vi "StartRotation.vi"(0 "Graphics Refnum in":refnum<k24>, 1 "X-In":sgl, 2 "Y-In":sgl, 3 "Width-In":sgl, 4 "Height-In":sgl, 5 "error in (no error)":errorcluster, 9 "Rotation(Deg)":sgl) -> (11 "dyTranslation":sgl, 13 "dxTranslation":sgl, 14 "Graphics Refnum out":refnum<k24>, 15 "X-Out":sgl, 16 "Y-Out":sgl, 17 "Width-Out":sgl, 18 "Height-Out":sgl, 19 "error out":errorcluster)   [LabVIEW 2020, in "LcPictureBox.lvclass"]
uses:
  <userlib>/_LabVIEWCommon/LcPictureBox_class/LcPictureBox.lvclass
  System.Drawing
  <userlib>/_LabVIEWCommon/LcPictureBox_class/LcPictureBox.lvclass/LcPictureBox.ctl
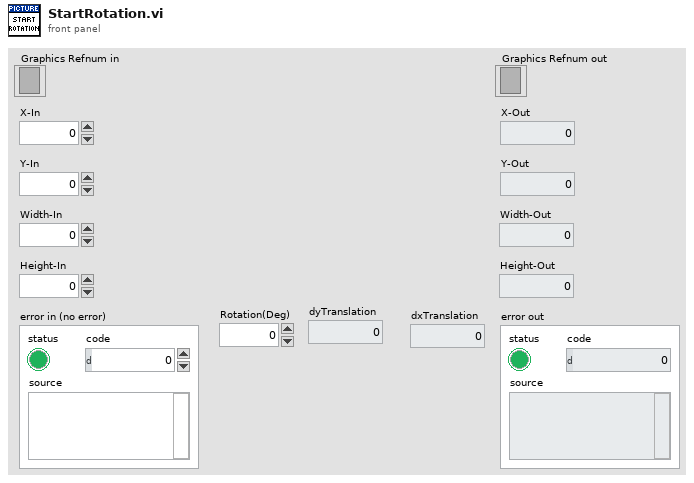
[diagram p1: front panel]
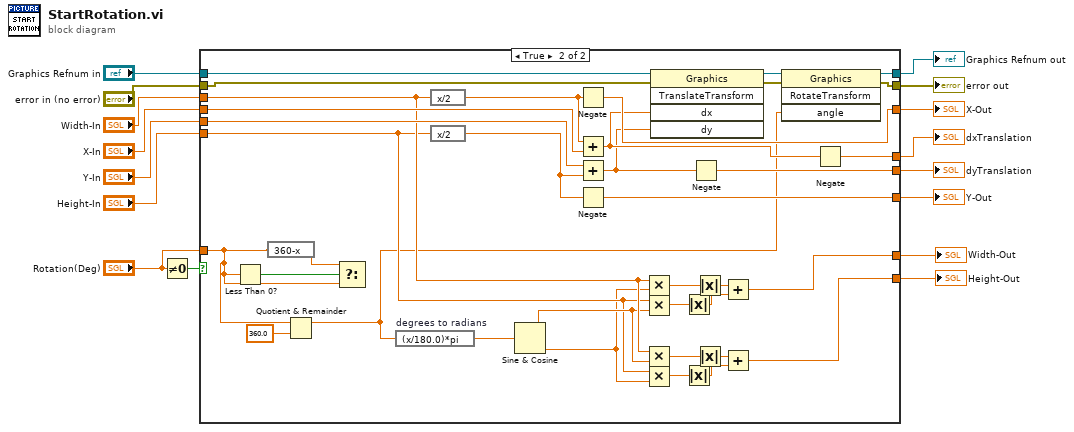
[diagram p0: block diagram]
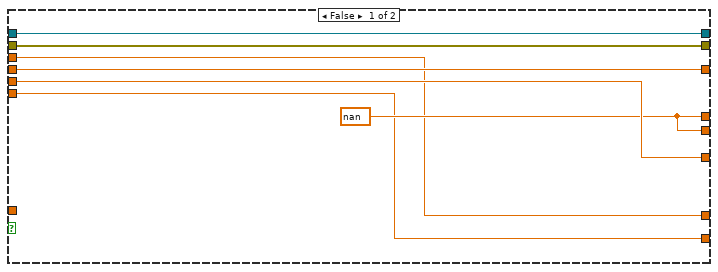
[diagram p2: hidden frame]
diagram:
  n1 = Not Equal To 0?(x="Rotation(Deg)") -> (x != 0?=w11:bool)
  n2 = case shown="True" w11 {
    tunnel: "Graphics Refnum in" -> [w23 w57]
    tunnel: [w23 w59] -> w8
    tunnel: "Rotation(Deg)" -> [_ w25]
    tunnel: "error in (no error)" -> [w22 w56]
    tunnel: [w22 w58] -> w10
    tunnel: [w21 w53] -> w6
    tunnel: [w20 w52] -> w5
    tunnel: "X-In" -> [w21 w51]
    tunnel: "Width-In" -> [w18 w37]
    tunnel: [w19 w49] -> w4
    tunnel: "Y-In" -> [w20 w48]
    tunnel: [w19 w46] -> w3
    tunnel: "Height-In" -> [w17 w35]
    tunnel: [w17 w33] -> w2
    tunnel: [w18 w40] -> w1
    frame False {
      w19 = sgl nan
    }
    frame True {
      n3 = Less Than 0?(x=w25) -> (x < 0?=w28:bool)
      n4 = expression code="360-x"(w25) -> (w27:sgl)
      n5 = Quotient & Remainder(x=w25, y=360.0) -> (x-y*floor(x/y)=w24:dbl)  [unwired: 1 out]
      n6 = Select(t=w27, s=w28, f=w25) -> ()  [unwired: 1 out]
      n7 = expression code="(x/180.0)*pi" "degrees to radians"(w24) -> (w43:dbl)
      n8 = expression code="x/2"(w37) -> (w45:sgl)
      n9 = expression code="x/2"(w35) -> (w44:sgl)
      n10 = Sine & Cosine(0:w43) -> (1:w36:dbl, 2:w34:dbl)
      n11 = Negate(x=w45) -> (-x=w53:sgl)
      n12 = Add(x=w45, y=w51) -> (x+y=w50:sgl)
      n13 = Add(x=w48, y=w44) -> (x+y=w47:sgl)
      n14 = Negate(x=w44) -> (-x=w52:sgl)
      n15 = Multiply(x=w37, y=w34) -> (x*y=w42:dbl)
      n16 = Multiply(x=w35, y=w36) -> (x*y=w41:dbl)
      n17 = Multiply(x=w37, y=w36) -> (x*y=w38:dbl)
      n18 = Multiply(x=w35, y=w34) -> (x*y=w39:dbl)
      n19 = invoke class="Graphics" method="TranslateTransform"(reference=w57, error in=w56, "dx"=w50, "dy"=w47) -> (reference out=w55:refnum<k24>, error out=w54:errorcluster)  [unwired: 1 in, 3 out]
      n20 = Absolute Value(x=w41) -> (abs(x)=w31:dbl)
      n21 = Absolute Value(x=w39) -> (abs(x)=w29:dbl)
      n22 = Negate(x=w47) -> (-x=w46:sgl)
      n23 = Absolute Value(x=w42) -> (abs(x)=w32:dbl)
      n24 = Absolute Value(x=w38) -> (abs(x)=w30:dbl)
      n25 = Add(x=w32, y=w31) -> (x+y=w40:dbl)
      n26 = Add(x=w30, y=w29) -> (x+y=w33:dbl)
      n27 = invoke class="Graphics" method="RotateTransform"(reference=w55, error in=w54, "angle"=w24) -> (reference out=w59:refnum<k24>, error out=w58:errorcluster)  [unwired: 1 in, 2 out]
      n28 = Negate(x=w50) -> (-x=w49:sgl)
    }
  }
  "error out" <- w10
  "Graphics Refnum out" <- w8
  "X-Out" <- w6
  "Y-Out" <- w5
  "dxTranslation" <- w4
  "dyTranslation" <- w3
  "Height-Out" <- w2
  "Width-Out" <- w1
